vi "KObjTemplate-Base-To Variant.vi"(0 "Obj in":refnum<class "KObject.lvclass">, 11 "error in (no error)":errorcluster) -> (4 "Obj out":refnum<class "KObject.lvclass">, 8 "Array":variant[](array[variant]), 15 "error out":errorcluster)   [LabVIEW 2015]
uses:
  KObject Class/KObject.lvclass
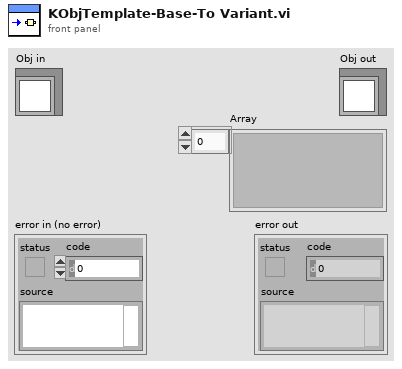
[diagram p1: front panel]
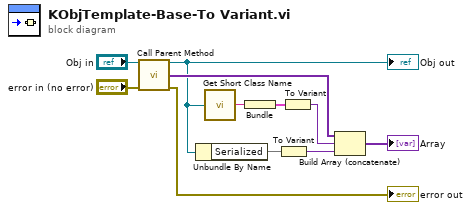
[diagram p0: block diagram]
diagram:
  n1 = call-parent "Call Parent Method"("KObject in"="Obj in", "error in (no error)"="error in (no error)") -> ("KObject out"=w4:refnum<class "TTLControlledDevice.lvclass">, "Array"=w7:variant[], "error out"=→"error out":errorcluster)  [unwired: 11 in]
  "Obj out" <- w4
  n2 = Unbundle By Name(w4) -> ("Serialized"=w8)
  n3 = call "Get Short Class Name.vi"("KObject in"=w4) -> ("Class"=w3:string)  [unwired: 4 in]
  n4 = Bundle("Class"=w3) -> (w2:cluster{"Class":string})  [unwired: 1 in]
  n5 = To Variant(anything=w8) -> (Variant=w5:variant)
  n6 = To Variant(anything=w2) -> (Variant=w1:variant)
  n7 = Build Array (concatenate)(w7, w1, w5) -> (→"Array":variant[])
